vi "CFTS-Terminal Configuration Dialog.vi"(2 "Parent VI":refnum<vi>) -> ()   [LabVIEW 2020]
doc: "Use this template to create a dialog box with event handling."
uses:
  epl-vi-lib/Utility VIs/Controls/KBackground Gradient/KBackground Gradient.xctl
  epl-vi-lib/Utility VIs/Controls/KTable/KTable.xctl
  epl-vi-lib/Utility VIs/File IO VIs/Configuration File Wrapper VIs/Config-Write Key (string).vi
panel:
  in  "AO":u16(xcontrol)
  in  "AI":u16(xcontrol)
  in  "background":dbl(xcontrol)
  in  "Cancel":bool
  in  "OK":bool
  # "Terminal configuration"
  # "Outputs"
  # "Inputs"
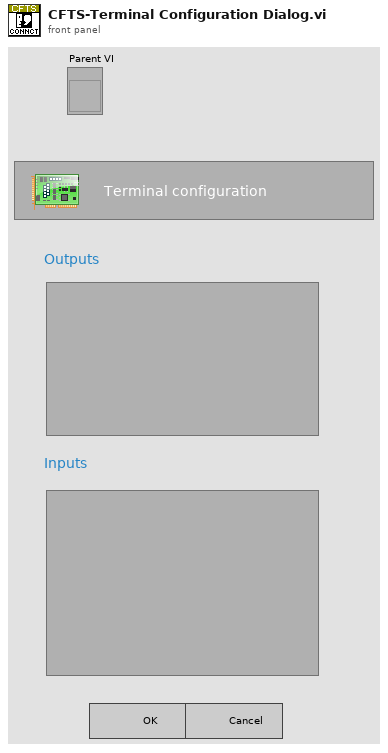
[diagram p1: front panel]
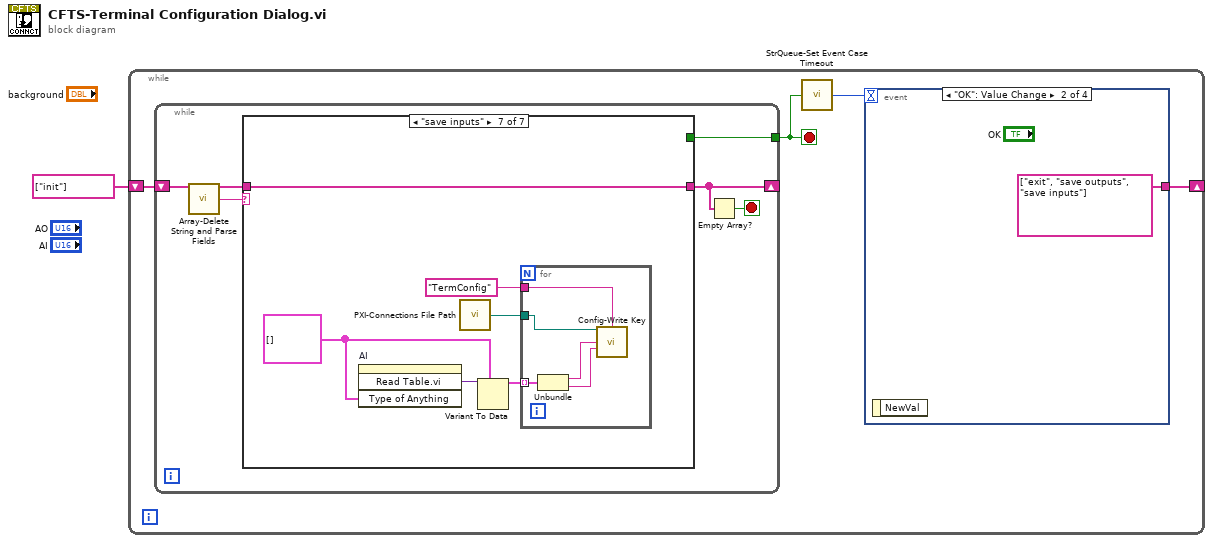
[diagram p0: block diagram]
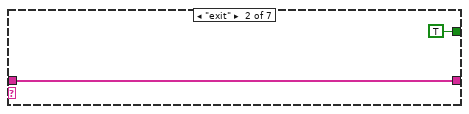
[diagram p3: hidden frame]
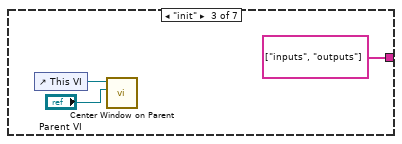
[diagram p4: hidden frame]
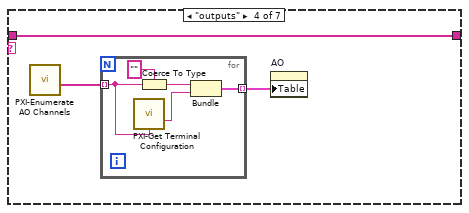
[diagram p5: hidden frame]
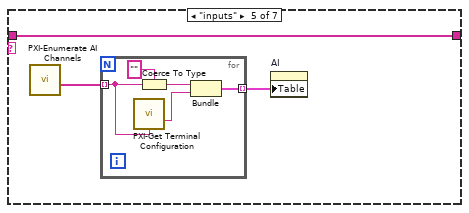
[diagram p6: hidden frame]
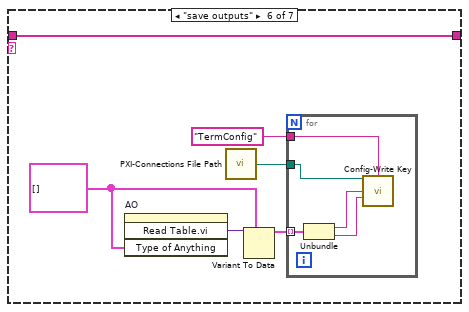
[diagram p7: hidden frame]
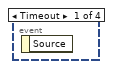
[diagram p8: hidden frame]
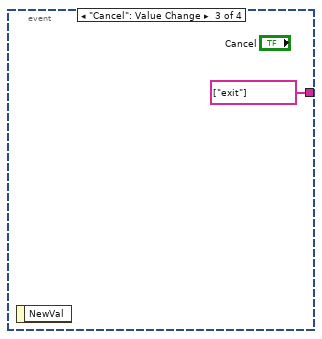
[diagram p9: hidden frame]
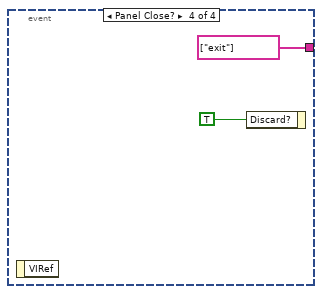
[diagram p10: hidden frame]
diagram:
  n1 = while {
    shift-right: [w2] -> _
    shift-left: string[] ["init"] -> [w3]
    stop <- w5 stop-if-true
    n2 = while {
      shift-right: [w11] -> _
      shift-left: w3 -> [w8]
      tunnel: [w9] -> w5
      stop <- w10 stop-if-true
      n3 = call "Array-Delete String and Parse Fields.vi"("Array in"=w8) -> ("Array out"=w7:string[], "Field 1"=w6:string)  [unwired: 10 in, 3 out]
      n4 = case shown="\"save inputs\"" w6 {
        tunnel: w7 -> [w12 w14 _ w20 w28 w39 w50]
        tunnel: [w12 w14 string[] ["inputs", "outputs"] ("Array out") w20 w28 w39 w50] -> w11
        tunnel: [_ TRUE _ _ _ _ _] -> w9
        frame "", Default {
        }
        frame "exit" {
        }
        frame "init" {
          n5 = control-ref of="This VI"() -> (w16:refnum<vi>)
          n6 = call "Center Window on Parent.vi"("Parent VI"="Parent VI", "VI in"=w16) -> ()  [unwired: 8 in, 2 out]
        }
        frame "outputs" {
          n7 = call "PXI-Enumerate AO Channels.vi"() -> ("24-bit channels"=w19:tag[])  [unwired: 10 in, 1 out]
          n8 = for {
            tunnel: w19 -> [w24] mode=indexing
            tunnel: [w25] -> w18 mode=indexing
            n9 = call "PXI-Get Terminal Configuration.vi"("channel"=w24) -> ("term config name"=w21:string)  [unwired: 12 in, 2 out]
            n10 = Coerce To Type(0:w24, 1:"") -> (2:w22:string)
            n11 = Bundle(w22, "term config name"=w21) -> (w25:cluster{string, "term config name":string})  [unwired: 1 in]
          }
          n12 = property on="AO" class="KTable (strict)"("Table"=w18) -> ()  [unwired: 2 in, 2 out]
        }
        frame "inputs" {
          n13 = call "PXI-Enumerate AI Channels.vi"() -> ("24-bit channels"=w26:tag[])  [unwired: 10 in, 1 out]
          n14 = for {
            tunnel: w26 -> [w32] mode=indexing
            tunnel: [w33] -> w27 mode=indexing
            n15 = call "PXI-Get Terminal Configuration.vi"("channel"=w32) -> ("term config name"=w29:string)  [unwired: 12 in, 2 out]
            n16 = Coerce To Type(0:w32, 1:"") -> (2:w30:string)
            n17 = Bundle(w30, "term config name"=w29) -> (w33:cluster{string, "term config name":string})  [unwired: 1 in]
          }
          n18 = property on="AI" class="KTable (strict)"("Table"=w27) -> ()  [unwired: 2 in, 2 out]
        }
        frame "save outputs" {
          w37 = cluster{string, string}[] [] ("Array")
          n19 = invoke on="AO" class="KTable (strict)" method="Read Table.vi"("Type of Anything"=w37) -> ("Read Table.vi"=w38:variant)  [unwired: 3 in, 3 out]
          n20 = call "PXI-Connections File Path.vi"() -> ("Path"=w36:path)  [unwired: 1 in]
          n21 = Variant To Data(type=w37, Variant=w38) -> (data=w34:cluster{string, string}[])  [unwired: 1 in, 1 out]
          n22 = for {
            tunnel: w36 -> [w44]
            tunnel: "TermConfig" ("section") -> [w43]
            tunnel: w34 -> [w42] mode=indexing
            n23 = Unbundle(w42) -> (w41:string, w40:string)
            n24 = call-poly "Config-Write Key.vi"("configuration file path"=w44, "section"=w43, "key"=w41, "value"=w40) -> ()  [unwired: 9 in, 3 out]
          }
        }
        frame "save inputs" {
          w48 = cluster{string, string}[] [] ("Array")
          n25 = invoke on="AI" class="KTable (strict)" method="Read Table.vi"("Type of Anything"=w48) -> ("Read Table.vi"=w49:variant)  [unwired: 3 in, 3 out]
          n26 = call "PXI-Connections File Path.vi"() -> ("Path"=w47:path)  [unwired: 1 in]
          n27 = Variant To Data(type=w48, Variant=w49) -> (data=w45:cluster{string, string}[])  [unwired: 1 in, 1 out]
          n28 = for {
            tunnel: w47 -> [w55]
            tunnel: "TermConfig" ("section") -> [w54]
            tunnel: w45 -> [w53] mode=indexing
            n29 = Unbundle(w53) -> (w52:string, w51:string)
            n30 = call-poly "Config-Write Key.vi"("configuration file path"=w55, "section"=w54, "key"=w52, "value"=w51) -> ()  [unwired: 9 in, 3 out]
          }
        }
      }
      n31 = Empty Array?(array=w11) -> (empty?=w10:bool)
    }
    n32 = call "StrQueue-Set Event Case Timeout.vi"("Quit"=w5) -> ("timeout"=w4:i32)  [unwired: 14 in]
    n33 = event shown="[1] \"OK\": Value Change" {
      selector: _ -> [_ _ _ _]
      dyn-events: _ -> [_ _ _ _]
      timeout: w4 -> [_ _ _ _]
      tunnel: [_ string[] ["exit", "save outputs", "save inputs"] string[] ["exit"] string[] ["exit"]] -> w2
      event Timeout {
        n34 = event-data() -> ()  [unwired: 1 in, 1 out]
      }
      event "OK": Value Change {
        n35 = event-data() -> ()  [unwired: 1 in, 1 out]
      }
      event "Cancel": Value Change {
        n36 = event-data() -> ()  [unwired: 1 in, 1 out]
      }
      event Panel Close? {
        n37 = event-data() -> ()  [unwired: 1 in, 1 out]
        n38 = event-data("Discard?"=TRUE) -> ()  [unwired: 1 in, 1 out]
      }
    }
  }
